vi "Init.vi"(8 "error in (no error)":errorcluster, 10 "Channel":i16, 11 "TrialBasedExperiment in":refnum<class "PassiveFixation.lvclass">) -> (0 "error out":errorcluster, 3 "TrialBasedExperiment out":refnum<class "PassiveFixation.lvclass">)   [LabVIEW 2010, in "PassiveFixation.lvclass"]
doc: "Author: Mani Subramaniyan\nDate: 2011-09-06"
uses:
  PassiveFixation.lvclass
  PassiveExperiment/PassiveExperiment.lvclass
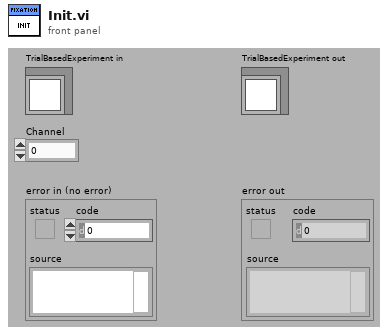
[diagram p1: front panel]
types:
  T1 = cluster{"Intertrial":dbl, "AcquireFixation":dbl, "HoldFixation":dbl, "DelayPeriod":dbl, "ResponsePeriod":dbl}
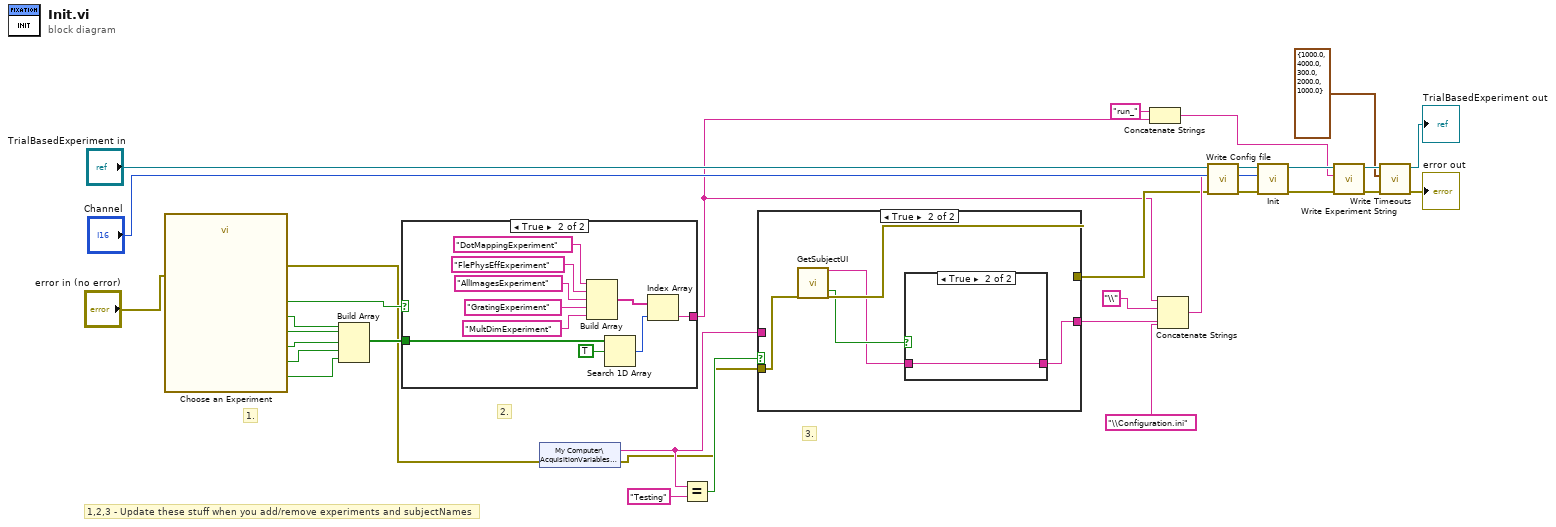
[diagram p0: block diagram]
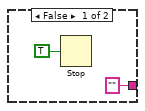
[diagram p3: hidden frame]
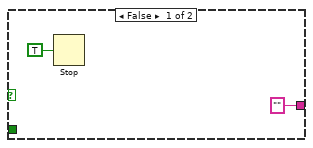
[diagram p4: hidden frame]
diagram:
  # "1,2,3 - Update these stuff when you add/remove experiments and subjectNames"
  # "3."
  # "2."
  # "1."
  n1 = call "Choose an Experiment"("error in (no error)"="error in (no error)") -> ("MultDimExperiment"=w4:bool, "GratingExperiment"=w24:bool, "AllImagesExperiment"=w25:bool, "FlePhysEffExperiment"=w26:bool, "DotMappingExperiment"=w27:bool, "OK"=w23:bool, "error out"=w5:errorcluster)  [unwired: 12 in]
  n2 = Build Array(w27, w26, w25, w24, w4) -> (w22:bool[])
  n3 = case shown="True" w23 {
    tunnel: w22 -> [_ w39]
    tunnel: ["" w36] -> w3
    frame False {
      n4 = Stop(stop? (T)=TRUE) -> ()
    }
    frame True {
      n5 = Build Array("DotMappingExperiment", "FlePhysEffExperiment", "AllImagesExperiment", "GratingExperiment", "MultDimExperiment") -> (w38:string[])
      n6 = Search 1D Array(1D array=w39, element=TRUE) -> (index of element=w37:i32)  [unwired: 1 in]
      n7 = Index Array(array=w38, index=w37) -> (element=w36:string)
    }
  }
  n8 = shared-variable "My Computer\\AcquisitionVariables.lvlib\\Subject"(error in=w5) -> (w10:string, error out=w9:errorcluster)
  n9 = Equal?(x=w10, y="Testing") -> (x = y?=w12:bool)
  n10 = case shown="True" w12 {
    tunnel: [w46 w47] -> w7
    tunnel: w10 -> [w46 _]
    tunnel: w9 -> [w45 w51]
    tunnel: [w45 w50] -> w8
    frame False {
    }
    frame True {
      n11 = call "GetSubjectUI.vi"("error in (no error)"=w51) -> ("subjectSelected"=w48:string, "OK"=w49:bool, "error out"=w50:errorcluster)  [unwired: 16 in]
      n12 = case shown="True" w49 {
        tunnel: w48 -> [_ w54]
        tunnel: ["" ("subjectSelected") w54] -> w47
        frame False {
          n13 = Stop(stop? (T)=TRUE) -> ()
        }
        frame True {
        }
      }
    }
  }
  n14 = Concatenate Strings("run_" ("string"), w3) -> (w1:string)
  n15 = Concatenate Strings(w3, "\\", w7, "\\Configuration.ini") -> (w21:string)
  n16 = call-dynamic "Write Config file.vi"("error in (no error)"=w8, "Config file"=w21, "TrialBasedExperiment in"="TrialBasedExperiment in") -> ("error out"=w15:errorcluster, "TrialBasedExperiment out"=w17:refnum<class "PassiveFixation.lvclass">)  [unwired: 7 in]
  n17 = call-parent "Init.vi"("error in (no error)"=w15, "Channel"="Channel", "TrialBasedExperiment in"=w17) -> ("error out"=w19:errorcluster, "TrialBasedExperiment out"=w20:refnum<class "PassiveFixation.lvclass">)  [unwired: 7 in]
  n18 = call-dynamic "Write Experiment String.vi"("error in (no error)"=w19, "Experiment String"=w1, "TrialBasedExperiment in"=w20) -> ("error out"=w29:errorcluster, "TrialBasedExperiment out"=w31:refnum<class "PassiveFixation.lvclass">)  [unwired: 7 in]
  n19 = call-dynamic "Write Timeouts.vi"("error in (no error)"=w29, "Timeouts"=T1 {"Intertrial"=1000.0, "AcquireFixation"=4000.0, "HoldFixation"=300.0, "DelayPeriod"=2000.0, "ResponsePeriod"=1000.0}, "TrialBasedExperiment in"=w31) -> ("error out"=→"error out":errorcluster, "TrialBasedExperiment out"=→"TrialBasedExperiment out":refnum<class "PassiveFixation.lvclass">)  [unwired: 7 in]
